vi "数字波形.vi"() -> ()   [LabVIEW 2010]
uses:
  <vilib>/Analysis/NI_AALBase.lvlib
panel:
  out "Digital Waveform":digitalwaveform(waveform)
  in  "最大值":dbl=1.0
  in  "最小值":dbl=-1.0
  in  "分辨率":i32=16
  in  "信号幅值":dbl=1.0 format="%0.2f"
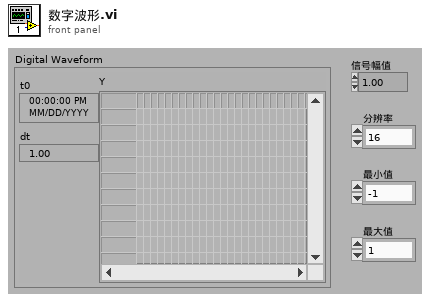
[diagram p1: front panel]
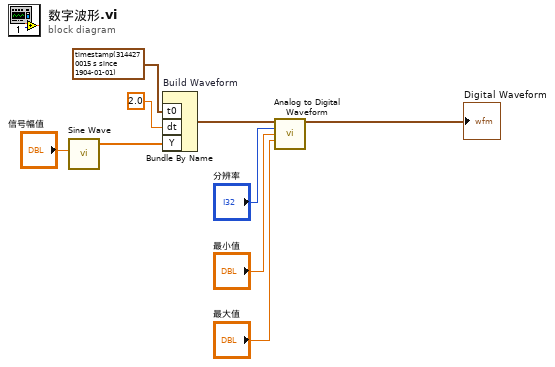
[diagram p0: block diagram]
diagram:
  n1 = call <vilib>:"Sine Wave.vi"("amplitude"="信号幅值") -> ("sine wave"=w8:dbl[])  [unwired: 4 in, 2 out]
  n2 = Bundle By Name "Build Waveform"("t0"=timestamp(3144270015 s since 1904-01-01), "dt"=2.0, "Y"=w8) -> (w6:waveform(dbl))  [unwired: 1 in]
  n3 = call <vilib>:"Analog to Digital Waveform.vi"("Analog Waveform"=w6, "Resolution (16 bit)"="分辨率", "Min (-1.0)"="最小值", "Max (1.0)"="最大值") -> ("Digital Waveform"=→"Digital Waveform":digitalwaveform)  [unwired: 7 in, 4 out]
